vi "play_FXP_AFM_MIMO_MPC.vi"() -> ()   [LabVIEW 2017]
uses:
  <vilib>/rvi/interface/nirviMethod/nirviMethod.xnode
  <vilib>/rvi/errors/niLvFpgaMergeErrorWithErrorCode.vi
  <vilib>/rvi/interface/nirviReadWriteControl/nirviReadWriteControl.xnode
  <vilib>/rvi/errors/niLvFpgaAdjustHostInterfaceError.vi
  <vilib>/Utility/file.llb/Write To Spreadsheet File (DBL).vi
  <vilib>/rvi/interface/nirviOpenFPGA/nirviOpenFPGA.xnode
  <vilib>/userdefined/High Color/nirio_resource_hc.ctl
  <vilib>/FPGAPlugInAG/Dynamic/niLvFpga_Reset_Dynamic.vi
  <vilib>/rvi/interface/Simulation/niFpgaSimulationCallBeginRW.vi
  <vilib>/FPGAPlugInAG/Dynamic/niLvFpga_Run_Dynamic.vi
  <vilib>/FPGAPlugInAG/Dynamic/niLvFpga_ReadFifo_Dynamic.vi
  <vilib>/rvi/interface/nirviMethod/StockFPGA_InlinedMethodWaitForSingleIRQ.vi
  <vilib>/FPGAPlugInAG/Dynamic/niLvFpga_WaitOnIrq_Dynamic.vi
  <vilib>/FPGAPlugInAG/Dynamic/niLvFpga_AcknowledgeIrq_Dynamic.vi
  <vilib>/rvi/interface/nirviCloseFPGA/nirviCloseFPGA.xnode
  <vilib>/FPGAPlugInAG/Dynamic/niLvFpga_ConfigureFifo_Dynamic.vi
  FPGA Bitfiles/afmMPCmultiAxis_FPGATarget_FXPAFMssMPCmulti_axis.lvbitx
  <vilib>/FPGAPlugInAG/Dynamic/niLvFpga_WriteFifo_Dynamic.vi
  <vilib>/FPGAPlugInAG/Dynamic/niLvFpga_Close_Dynamic.vi
  <vilib>/FPGAPlugInAG/cRIO-9082/niLvFpga_Open_cRIO-9082.vi
  <vilib>/rvi/interface/common/dynamic/niFpgaDynamicAddResources.vi
  fpga_VIs/fixed-point/typeDefs/FXPControlParams_distEst.ctl
  controls/ObserverMatrices.ctl
  fpga_VIs/fixed-point/single-axis/fxp_mpc/fgm_pipiline/quadProgParams_pipe.ctl
panel:
  out "QP_params 2":T1={"maxIter"=0, "nuN"=24, "Ns_mpc"=0, "-beta"=-0.9987945556640625, "beta+1"=1.9987945556640625}
  out "ControlMatrices":T2
  out "MPC matrices":dbl[][](array[numeric])
  in  "Tab Control":enum32{"Page 1", "Page 2"}(tab)
  out "Actual Depth":u32
  out "FPGA_Diagnostics":T3
  out "u(k)Out":fxp<+/-,18,5>[](array[numeric])
  out "ControlParamsMpc":T4={"umax"=3.0, "NS"=0, "ref_f_VEC"=[0.0, 0.0], "du_max"=0.0}
  out "Empty Elements Remaining":u32
  out "Fifo matrix TimeOUt 2":bool
  out "Error Out 2":errorcluster
  out "Fifo matrix TimeOUt":bool
  out "Error Out":errorcluster
  out "y(0)":fxp<+/-,16,5>
  out "Stopped 2":bool
  out "yk_fast":fxp<+/-,16,5>
  out "error out":errorcluster
  out "yk to":bool
  out "Loop Ticks (benchmark)":i16
  out "WrteData":bool
  out "AI Timed Out":bool
  in  "Stop":bool
  in  "control_data_path":path=path "C:/Users/arnold/Documents/MATLAB/AFM_MPC/data/MPCControls01.csv"
  in  "outputDataPath":path=path "C:/Users/arnold/Documents/MATLAB/AFM_MPC/data/exp01outputBOTH.csv"
  in  "SettleTicks":i32=10
  out "y iter":i32
  out "size(s)":i32
  in  "Iters":i32=25
  in  "ymax":dbl=4.0 format="%#_13g"
  in  "umax":dbl=1.0 format="%#_13g"
  in  "TsTicks":i32=1600
  # "NOTE: Ns is the number of states in the plant. The number of states in the \nobserver is Ns+1. Thus, for B, L, C, and A, we use NS+1. For K and Xss, we use Ns\nbecause the controller does not operate on the disturbance state, Xd."
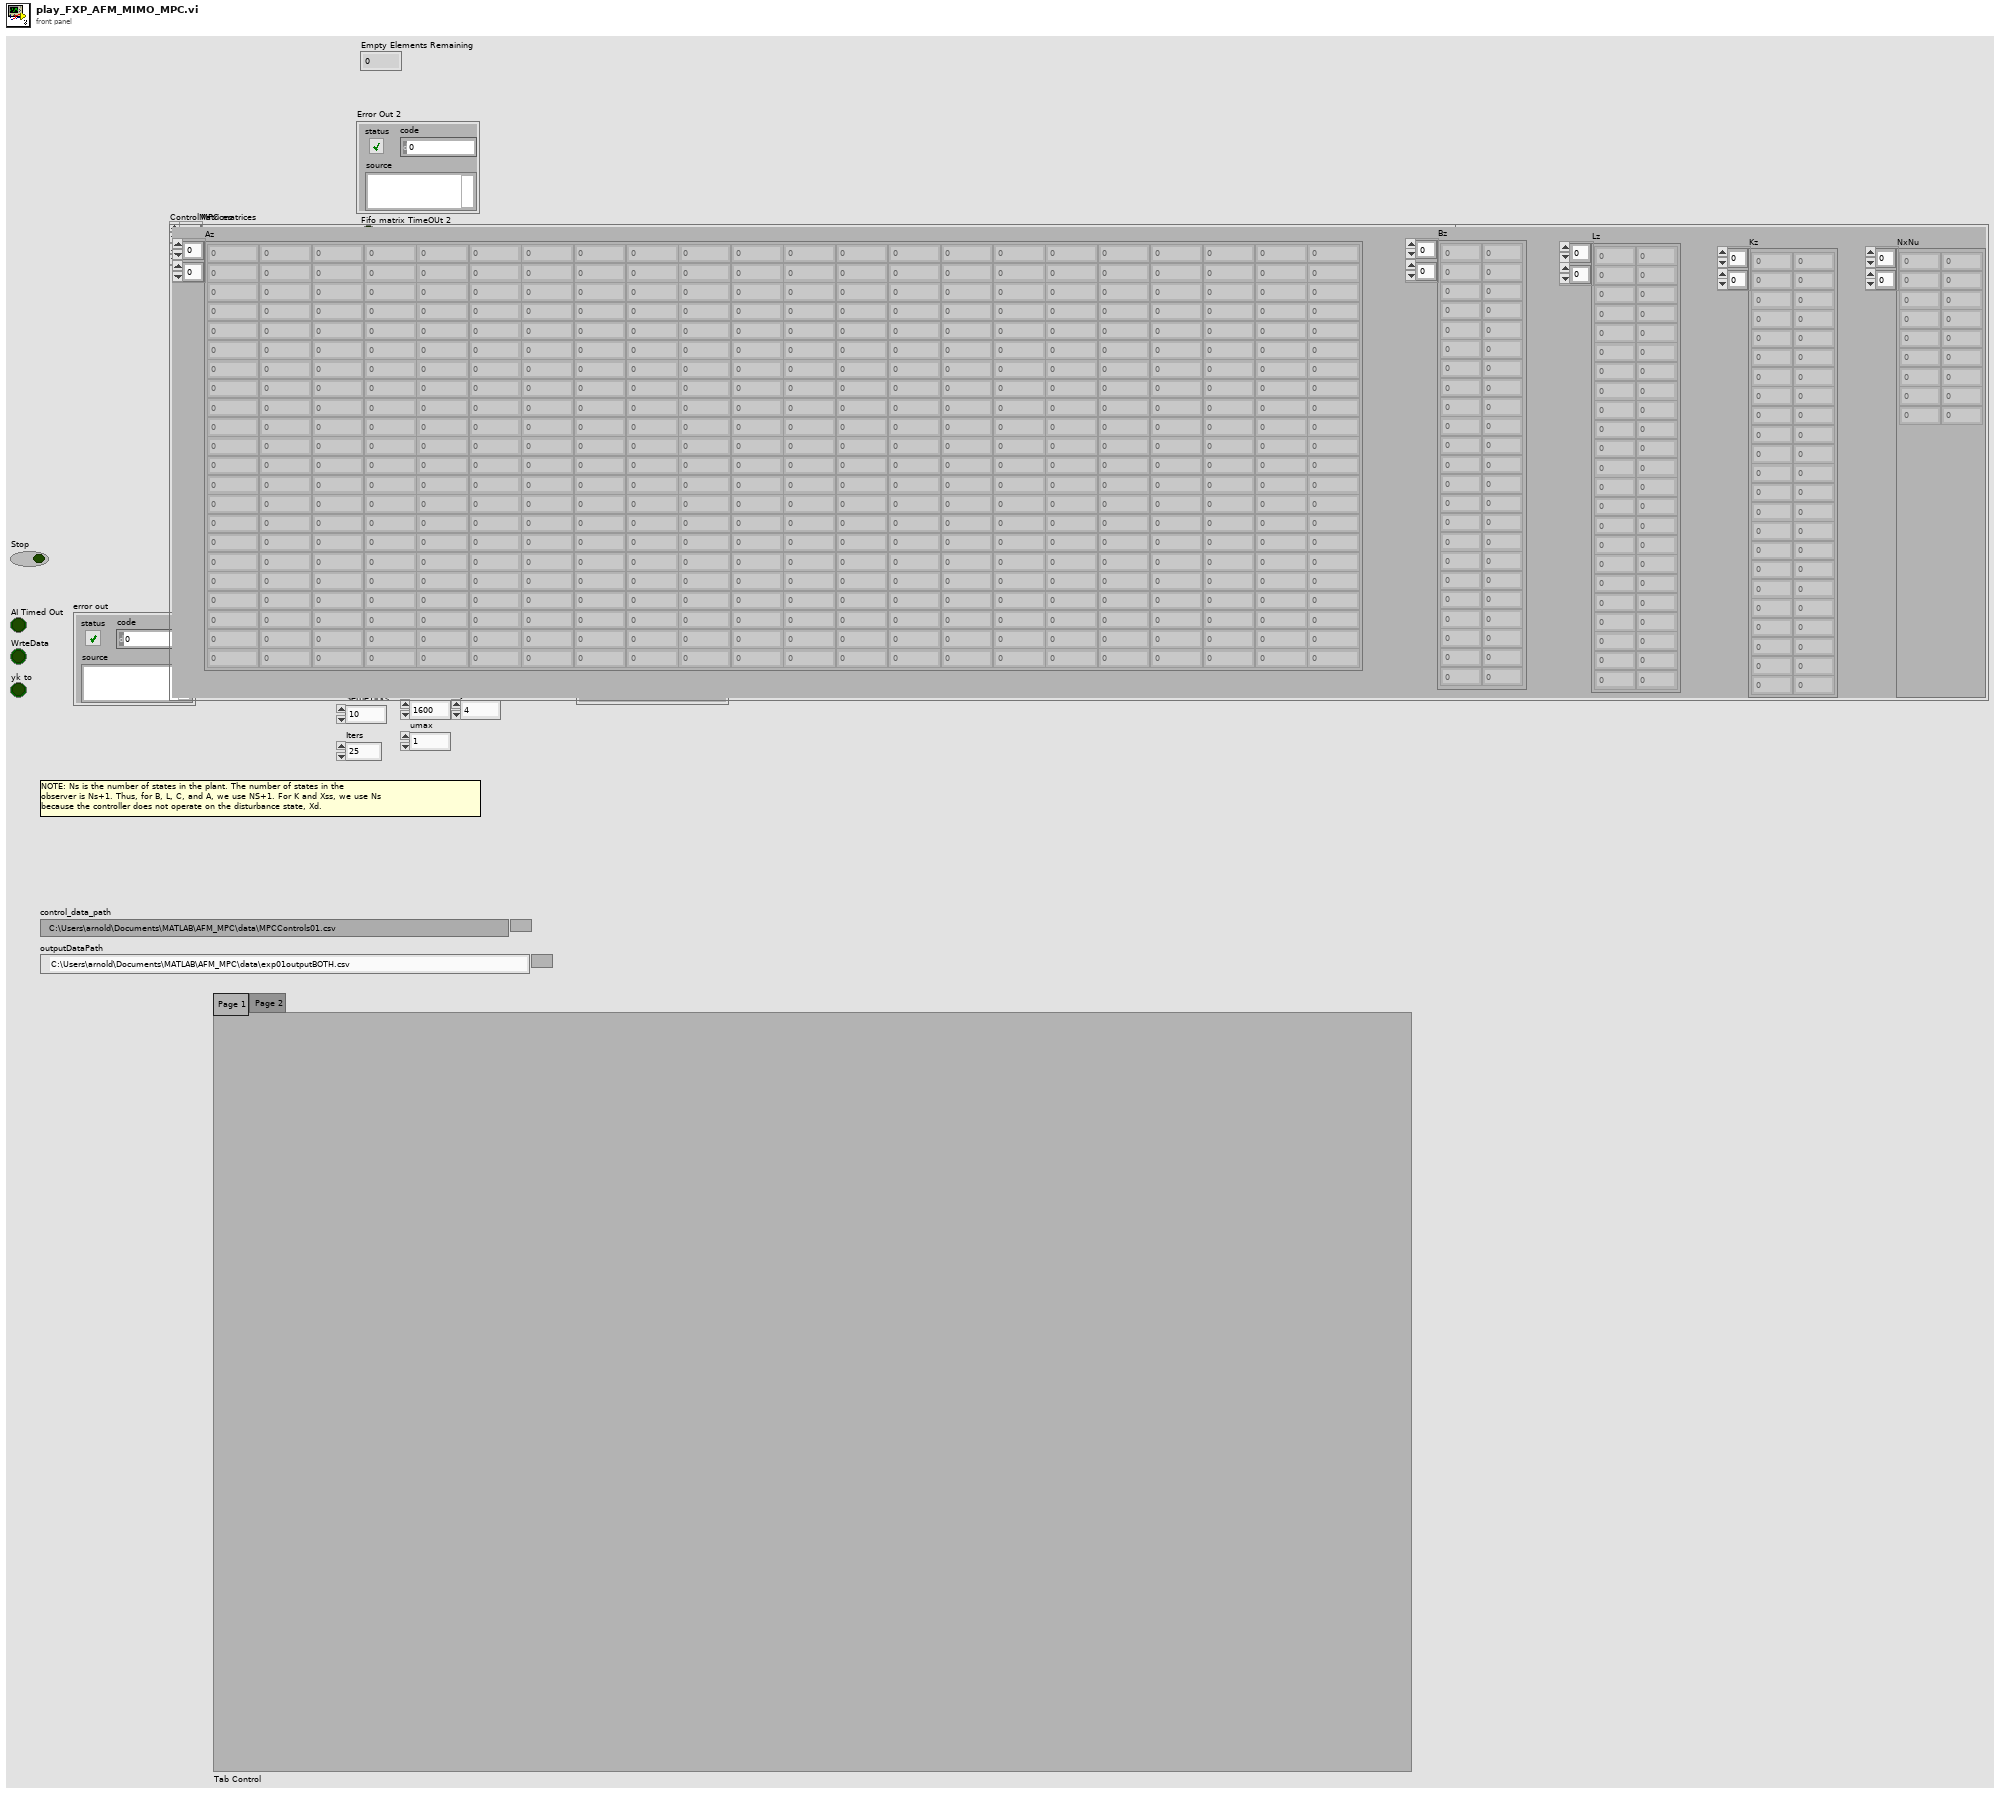
[diagram p1: front panel]
types:
  T1 = typedef "quadProgParams_pipe.ctl" = cluster{"maxIter":u16, "nuN":u16, "Ns_mpc":u16, "-beta":fxp<+/-,18,2>, "beta+1":fxp<+/-,18,2>}
  T2 = typedef "ObserverMatrices.ctl" = cluster{"Az":fxp<+/-,32,4>[][], "Bz":dbl[][], "Lz":dbl[][], "Kz":dbl[][], "NxNu":dbl[][]}
  T3 = cluster{"Y(k) Time Out":bool, "uxK Time Out":bool, "Unstable Trajes":bool[]}
  T4 = typedef "FXPControlParams_distEst.ctl" = cluster{"umax":fxp<+/-,18,5>, "NS":u8, "ref_f_VEC":fxp<+/-,32,5>[], "du_max":fxp<+/-,18,5>}
  T5 = typedef "nirio_resource_hc.ctl" = tag
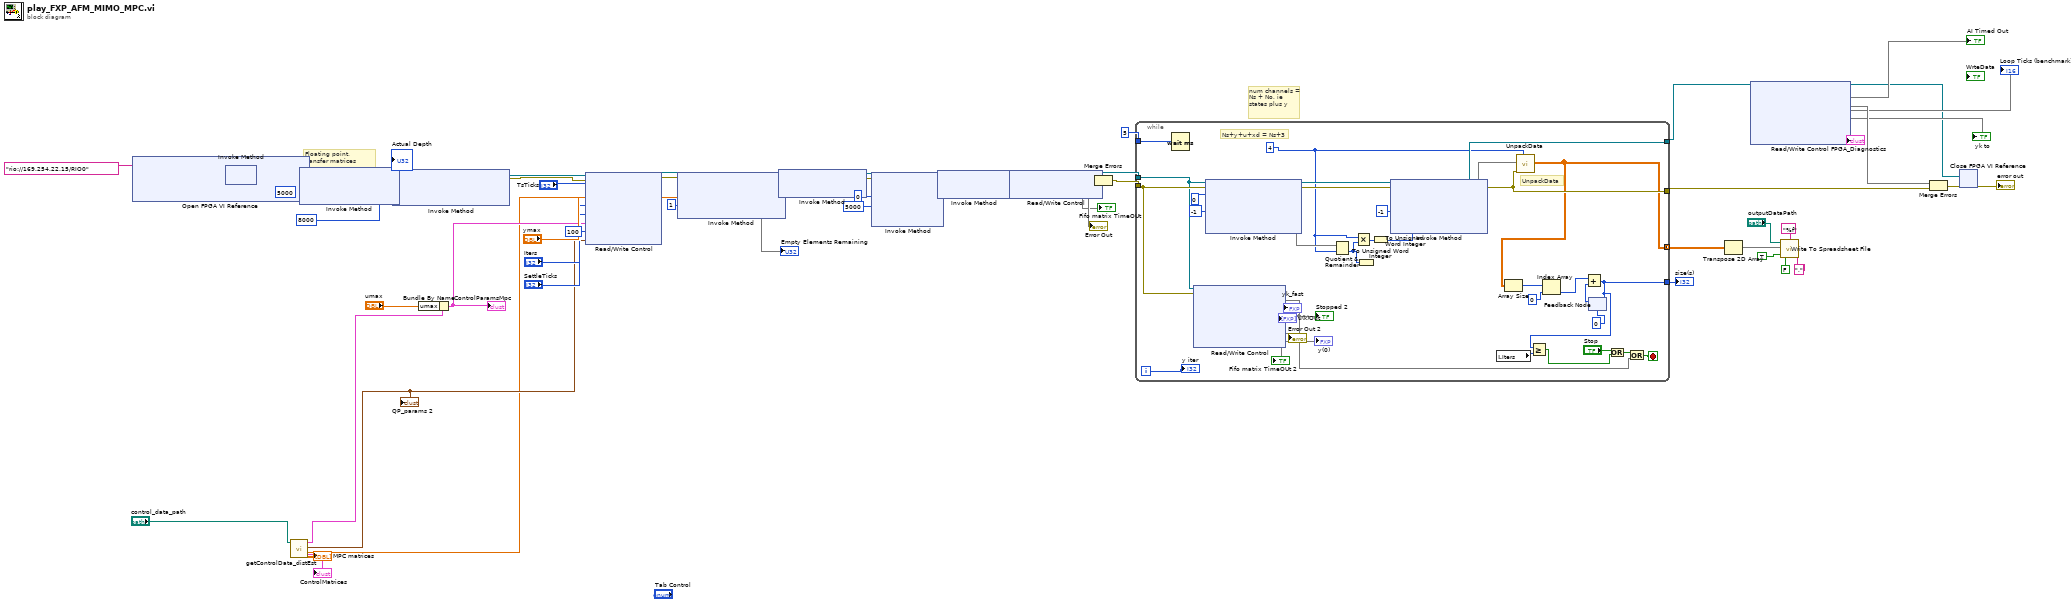
[diagram p0: block diagram]
diagram:
  # "Floating point, \ntransfer matrices"
  # "num channels = Ns + No, ie states plus y"
  n1 = xnode "Open FPGA VI Reference"("resource name"=T5 "rio://169.254.22.15/RIO0") -> ("FPGA VI Reference Out"=w49:refnum<k20>, "error out"=w53:errorcluster)  [unwired: 1 in]
  n2 = xnode "Invoke Method"("FPGA VI Reference In"=w49, "error in"=w53) -> ("FPGA VI Reference Out"=w47:refnum<k20>, "error out"=w46:errorcluster)
  n3 = call "getControlData_distEst.vi"("system matricec path"="control_data_path") -> ("MPC matrices"=→"MPC matrices":dbl[][], "AllMatrix"=w4:dbl[], "QP_params"=w5:T1, "ControlParams"=w6:T4, "ControlMatrices"=→"ControlMatrices":T2)  [unwired: 6 in]
  "QP_params 2" <- w5
  n4 = xnode "Invoke Method"("FPGA VI Reference In"=w47, "error in"=w46, "Requested Depth"=u32 5000) -> ("FPGA VI Reference Out"=w18:refnum<k20>, "error out"=w17:errorcluster, "Actual Depth"=→"Actual Depth")
  n5 = xnode "Invoke Method"("FPGA VI Reference In"=w18, "error in"=w17, "Requested Depth"=u32 8000) -> ("FPGA VI Reference Out"=w16:refnum<k20>, "error out"=w15:errorcluster)  [unwired: 1 out]
  n6 = Bundle By Name(cluster=w6, "umax"="umax") -> (w9:T4)
  "ControlParamsMpc" <- w9
  n7 = xnode "Read/Write Control"("FPGA VI Reference In"=w16, "error in"=w15, "TsTicks"="TsTicks", "ymax"="ymax", "iters"="Iters", "Settle Ticks"="SettleTicks", "ControlParamsMpc"=w9, "Max TsTicks"=u32 100, "QP_params"=w5) -> ("FPGA VI Reference Out"=w58:refnum<k20>, "error out"=w57:errorcluster)
  n8 = xnode "Invoke Method"("FPGA VI Reference In"=w58, "error in"=w57, "Data"=w4, "Timeout (ms)"=1) -> ("FPGA VI Reference Out"=w61:refnum<k20>, "error out"=w60:errorcluster, "Empty Elements Remaining"=→"Empty Elements Remaining")
  n9 = xnode "Invoke Method"("FPGA VI Reference In"=w61, "error in"=w60) -> ("FPGA VI Reference Out"=w37:refnum<k20>, "error out"=w38:errorcluster)  [unwired: 1 in]
  n10 = xnode "Invoke Method"("FPGA VI Reference In"=w37, "error in"=w38, "IRQ Number(s)"=0, "Timeout (ms)"=5000) -> ("FPGA VI Reference Out"=w43:refnum<k20>, "error out"=w44:errorcluster, "IRQ(s) Asserted"=w40:i32)  [unwired: 1 out]
  n11 = xnode "Invoke Method"("FPGA VI Reference In"=w43, "error in"=w44, "IRQ Number(s)"=w40) -> ("FPGA VI Reference Out"=w42:refnum<k20>, "error out"=w41:errorcluster)
  n12 = xnode "Read/Write Control"("FPGA VI Reference In"=w42, "error in"=w41) -> ("FPGA VI Reference Out"=w35:refnum<k20>, "error out"=w45:errorcluster, "Error Out"=w13, "Matrix FIFO  TimeOut"=→"Fifo matrix TimeOUt")
  "Error Out" <- w13
  n13 = Merge Errors(w45, w13) -> (w33:errorcluster)
  n14 = while {
    tunnel: 5 -> [w99]
    tunnel: w35 -> [w80]
    tunnel: w33 -> [w81]
    tunnel: [w91] -> w50
    tunnel: [w90] -> w32
    tunnel: [w79] -> w56 mode=concatenating
    tunnel: [w77] -> w55
    i -> [w78]
    stop <- w76 stop-if-true
    w65 = u8 4 ("x")
    # "Ns+y+u+xd = Ns+3"
    # "UnpackData"
    n15 = Wait (ms)(milliseconds to wait=w99) -> ()  [unwired: 1 out]
    n16 = xnode "Read/Write Control"("FPGA VI Reference In"=w80, "error in"=w81) -> ("Stopped"=w72, "y-axis fast"=→"yk_fast", "u(k)Out"=→"u(k)Out", "y(0)"=→"y(0)", "Error Out"=→"Error Out 2", "Matrix FIFO  TimeOut"=→"Fifo matrix TimeOUt 2")  [unwired: 2 out]
    "Stopped 2" <- w72
    n17 = xnode "Invoke Method"("FPGA VI Reference In"=w80, "error in"=w81, "Number of Elements"=0 ("Timeout (ms)"), "Timeout (ms)"=-1) -> ("FPGA VI Reference Out"=w95:refnum<k20>, "error out"=w96:errorcluster, "Elements Remaining"=w87)  [unwired: 1 out]
    n18 = Quotient & Remainder(x=w87, y=w65) -> (floor(x/y)=w89:u8)  [unwired: 1 out]
    n19 = Multiply(x=w65, y=w89) -> (x*y=w93:u8)
    n20 = To Unsigned Word Integer(number=w89) -> ()  [unwired: 1 out]
    n21 = To Unsigned Word Integer(number=w93) -> (unsigned 16bit integer=w69:u16)
    n22 = xnode "Invoke Method"("FPGA VI Reference In"=w95, "error in"=w96, "Number of Elements"=w69, "Timeout (ms)"=-1) -> ("FPGA VI Reference Out"=w90:refnum<k20>, "error out"=w91:errorcluster, "Data"=w86:void[])  [unwired: 1 out]
    n23 = local read "Iters"() -> (w88:i32)
    n24 = call "UnpackData.vi"("NumChannels"=w65, "error In"=w91, "1D Data In"=w86) -> ("2D Data Out"=w79:dbl[][])  [unwired: 7 in, 1 out]
    n25 = Array Size(array=w79) -> (size(s)=w85:i32[])
    n26 = Index Array(array=w85, index=0) -> (element=w83:i32)
    n27 = feedback #1(0) -> (w84:i32)
    n28 = Add(x=w83, y=w84) -> (x+y=w77:i32)
    n29 = Greater Or Equal?(x=w77, y=w88) -> (x >= y?=w73:bool)
    n30 = feedback-in #1(w77) -> ()
    n31 = Or(x="Stop", y=w73) -> (x .or. y?=w75:bool)
    n32 = Or(x=w75, y=w72) -> (x .or. y?=w76:bool)
    "y iter" <- w78
  }
  "size(s)" <- w55
  n33 = Transpose 2D Array(2D array=w56) -> (transposed array=w22:dbl[][])
  n34 = xnode "Read/Write Control"("FPGA VI Reference In"=w32) -> ("FPGA VI Reference Out"=w21:refnum<k20>, "AI Timed Out"=→"AI Timed Out", "Error Out"=w26, "Loop Ticks (benchmark)"=→"Loop Ticks (benchmark)", "YK TO"=→"yk to", "FPGA_Diagnostics"=→"FPGA_Diagnostics")  [unwired: 1 in, 2 out]
  n35 = call-poly <vilib>:"Write To Spreadsheet File.vi"("delimiter (\\t)"=",", "transpose? (no:F)"=TRUE, "format (%.3f)"="%f", "append to file? (new file:F)"=FALSE, "2D data"=w22, "file path (dialog if empty)"="outputDataPath") -> ()  [unwired: 2 in, 1 out]
  n36 = Merge Errors(w26, w50) -> (w20:errorcluster)
  n37 = xnode "Close FPGA VI Reference"("FPGA VI Reference In"=w21, "error in"=w20) -> ("error out"=→"error out":errorcluster)
